vi "Determine Packet Type.vi"(11 "Packet First Byte":u8 format="%08b") -> (3 "Packet Type":refnum<class "ControlPacket.lvclass">)   [LabVIEW 2013, in "MQTT_Control_Packets.lvlib" / "ControlPacket.lvclass"]
uses:
  ControlPacket.lvclass
  MQTT_311/MQTTVersion.lvclass
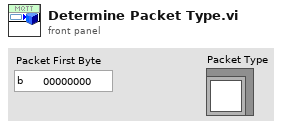
[diagram p1: front panel]
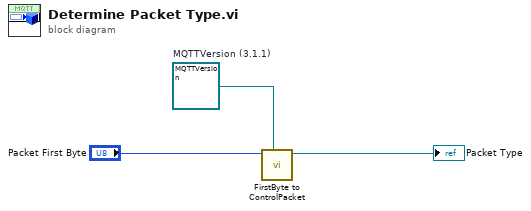
[diagram p0: block diagram]
diagram:
  w1 = refnum<class "MQTTVersion.lvclass"> refnum  # MQTTVersion (3.1.1)
  n1 = call-dynamic "FirstByte to ControlPacket.vi"("MQTTVersion"=w1, "Packet First Byte"="Packet First Byte") -> ("Packet Type"=→"Packet Type":refnum<class "ControlPacket.lvclass">)  [unwired: 9 in]
